vi "Convert_to_2009.vi"(8 "error in (no error)":errorcluster, 10 "2009 data in":T1={"DistSettings"={"BuildLabel"="", "ProductName"="", "BuildLocation"=path "", "MediaSize"=0, "Language"=9, "ProductVersion"={"Major"=1, "Minor"=0, "Update"=0}, "AutoIncrement"=FALSE, "ReadmeID"="", "LicenseID"="", "arpCompany"="", "arpURL"="http://", "arpContact"="", "arpPhone"="", "Executable"="", "CmdArg"="", "OSCheck"=0, "Hide"=FALSE, "LV80higher"=FALSE, "IncludeError?"=FALSE, "HWOption"=enum."<none>", "HWPath"=path "", "UpgradeCode"="", "Author"="", "MsiFileName"="", "CabFileName"="", "DistID"="", "WindowTitle"="", "WindowMessage"="", "CacheDistros"=FALSE, "EXE str ref?"=FALSE}, "BldInfo"=[], "FileInfo"=[], "DirInfo"=[], "ShortcutInfo"=[], "RegInfo"=[], "RegData"=[], "DistParts"=[], "DefaultDir"=""} {"RegData"."Values"."Type" items=["Bare", "String", "Expandable String", "Binary", "DWord"]; "DistSettings"."ProductVersion"."Update" step=1; "DistSettings"."ProductVersion"."Minor" step=1; "DistSettings"."ProductVersion"."Major" step=1; "DistSettings"."Language" items=["English"=9, "German"=7, "French"=12, "Japanese"=17, "Korean"=18, "Chinese (Simplified)"=2052]}, 11 "IB_Source_Build in":refnum<class "IB_Source_Build.lvclass">) -> (0 "error out":errorcluster, 2 "2009 data out":T1={"DistSettings"={"BuildLabel"="", "ProductName"="", "BuildLocation"=path "", "MediaSize"=0, "Language"=9, "ProductVersion"={"Major"=1, "Minor"=0, "Update"=0}, "AutoIncrement"=FALSE, "ReadmeID"="", "LicenseID"="", "arpCompany"="", "arpURL"="http://", "arpContact"="", "arpPhone"="", "Executable"="", "CmdArg"="", "OSCheck"=0, "Hide"=FALSE, "LV80higher"=FALSE, "IncludeError?"=FALSE, "HWOption"=enum."<none>", "HWPath"=path "", "UpgradeCode"="", "Author"="", "MsiFileName"="", "CabFileName"="", "DistID"="", "WindowTitle"="", "WindowMessage"="", "CacheDistros"=FALSE, "EXE str ref?"=FALSE}, "BldInfo"=[], "FileInfo"=[], "DirInfo"=[], "ShortcutInfo"=[], "RegInfo"=[], "RegData"=[], "DistParts"=[], "DefaultDir"=""} {"RegData"."Values"."Type" items=["Bare", "String", "Expandable String", "Binary", "DWord"]; "DistSettings"."ProductVersion"."Update" step=1; "DistSettings"."ProductVersion"."Minor" step=1; "DistSettings"."ProductVersion"."Major" step=1; "DistSettings"."Language" items=["English"=9, "German"=7, "French"=12, "Japanese"=17, "Korean"=18, "Chinese (Simplified)"=2052]})   [LabVIEW 2020, in "IB_Source_Build.lvclass"]
uses:
  <vilib>/AppBuilder/IB_Classes/Source/Container/Build/IB_Source_Build.lvclass
  <vilib>/AppBuilder/IB_Classes/Source/Container/Build/IB_Source_Build.lvclass/IB_Source_Build.ctl
  <vilib>/AppBuilder/IB_Classes/Source/IB_Source.lvclass
  <resource>/Framework/Providers/Builds/Installer/CDK_sTypeDef_BuildInfo.ctl
  <vilib>/AppBuilder/IB_Classes/Source/Container/IB_Source_Container.lvclass
  <resource>/Framework/Providers/Builds/Installer/CDK_sTypeDef_BuildTypes.ctl
  <vilib>/AppBuilder/IB_Classes/Source/File/IB_Source_File.lvclass
  e:/builds/penguin/labview/branches/2020/dev/dist/vi.lib/AppBuilder/IB_Classes/Source/Container/IB_Source_Container.lvclass
  e:/builds/penguin/labview/branches/2020/dev/dist/vi.lib/AppBuilder/IB_Classes/Source/IB_Source.lvclass
  e:/builds/penguin/labview/branches/2020/dev/dist/vi.lib/AppBuilder/IB_Classes/Source/Container/Build/IB_Source_Build.lvclass
  <vilib>/AppBuilder/IB_Classes/Source/File/CtrFile/IB_CtrFile.lvclass
  e:/builds/penguin/labview/branches/2020/dev/dist/vi.lib/AppBuilder/IB_Classes/Source/File/IB_Source_File.lvclass
  e:/builds/penguin/labview/branches/2020/dev/dist/vi.lib/AppBuilder/IB_Classes/Source/File/CtrFile/IB_CtrFile.lvclass
  <resource>/Framework/Providers/Builds/Installer/CDK_sTypeDef_FileInfo.ctl
  <resource>/Framework/Providers/Builds/Installer/CDK_sTypeDef_ShortcutInfo.ctl
  <resource>/Framework/Providers/Builds/Installer/CDK_sTypeDef_DirInfo.ctl
  <resource>/Framework/Providers/Builds/Installer/CDK_sTypeDef_Languages.ctl
  <resource>/Framework/Providers/Builds/Installer/CDK_sTypeDef_ProductVersion.ctl
  <resource>/Framework/Providers/Builds/Installer/CDK_sTypeDef_HWImportOption.ctl
  <resource>/Framework/Providers/Builds/Installer/CDK_sTypeDef_DISTSETTINGS.ctl
  AppLibs/distkit/MDF/NIMdf.llb/MDFBDPRegKeyType.ctl
  AppLibs/distkit/MDF/NI_MDF.lvlib
  <resource>/Framework/Providers/Builds/Installer/CDK_sTypeDef_RegData.ctl
  <resource>/Framework/Providers/Builds/Installer/CDK_sTypeDef_DistParts.ctl
  <vilib>/AppBuilder/IB_RW_Project/Compatibility/CDK_sTypeDef_2009_data.ctl
  <resource>/Framework/Providers/Builds/Installer/CDK_sTypeDef_SoftDep.ctl
panel:
  # "."
  # "."
  # "."
  # "."
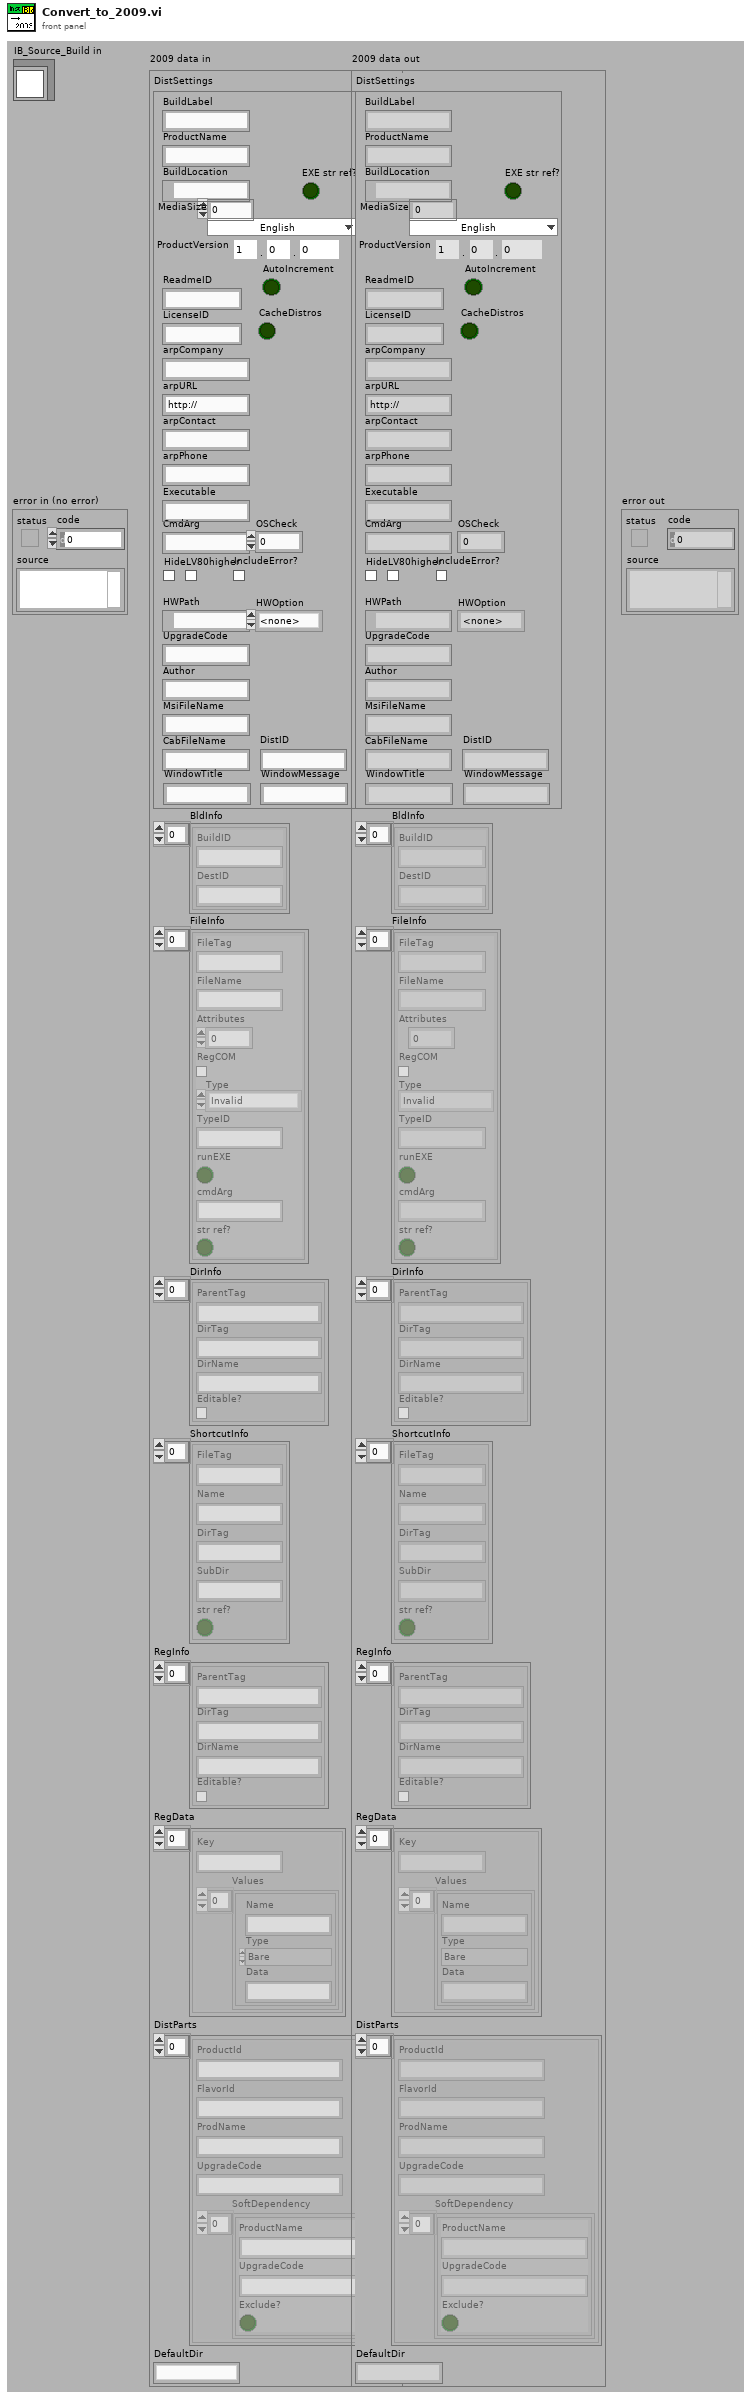
[diagram p1: front panel]
types:
  T1 = typedef "CDK_sTypeDef_2009_data.ctl" = cluster{"DistSettings":T2, "BldInfo":T6[], "FileInfo":T7[], "DirInfo":T9[], "ShortcutInfo":T10[], "RegInfo":T9[], "RegData":T11[], "DistParts":T13[], "DefaultDir":string}
  T2 = typedef "CDK_sTypeDef_DISTSETTINGS.ctl" = cluster{"BuildLabel":string, "ProductName":string, "BuildLocation":path, "MediaSize":u16, "Language":T3, "ProductVersion":T4, "AutoIncrement":bool, "ReadmeID":string, "LicenseID":string, "arpCompany":string, "arpURL":string, "arpContact":string, "arpPhone":string, "Executable":string, "CmdArg":string, "OSCheck":i32, "Hide":bool, "LV80higher":bool, "IncludeError?":bool, "HWOption":T5, "HWPath":path, "UpgradeCode":string, "Author":string, "MsiFileName":string, "CabFileName":string, "DistID":string, "WindowTitle":string, "WindowMessage":string, "CacheDistros":bool, "EXE str ref?":bool}
  T3 = typedef "CDK_sTypeDef_Languages.ctl" = u16
  T4 = typedef "CDK_sTypeDef_ProductVersion.ctl" = cluster{"Major":u8, "Minor":u8, "Update":u16}
  T5 = typedef "CDK_sTypeDef_HWImportOption.ctl" = enum16{"<none>", "Merge", "Replace", "Dialog"}
  T6 = typedef "CDK_sTypeDef_BuildInfo.ctl" = cluster{"BuildID":string, "DestID":string}
  T7 = typedef "CDK_sTypeDef_FileInfo.ctl" = cluster{"FileTag":string, "FileName":string, "Attributes":i16, "RegCOM":bool, "Type":T8, "TypeID":string, "runEXE":bool, "cmdArg":string, "str ref?":bool}
  T8 = typedef "CDK_sTypeDef_BuildTypes.ctl" = enum16{"Invalid", "File", "Folder", "BuildRule", "Library"}
  T9 = typedef "CDK_sTypeDef_DirInfo.ctl" = cluster{"ParentTag":string, "DirTag":string, "DirName":string, "Editable?":bool}
  T10 = typedef "CDK_sTypeDef_ShortcutInfo.ctl" = cluster{"FileTag":string, "Name":string, "DirTag":string, "SubDir":string, "str ref?":bool}
  T11 = typedef "CDK_sTypeDef_RegData.ctl" = cluster{"Key":string, "Values":cluster{"Name":string, "Type":T12, "Data":string}[]}
  T12 = typedef "NI_MDF.lvlib/MDFBDPRegKeyType.ctl" = i32
  T13 = typedef "CDK_sTypeDef_DistParts.ctl" = cluster{"ProductId":string, "FlavorId":string, "ProdName":string, "UpgradeCode":string, "SoftDependency":T14[]}
  T14 = typedef "CDK_sTypeDef_SoftDep.ctl" = cluster{"ProductName":string, "UpgradeCode":string, "Exclude?":bool}
  T15 = typedef "IB_Source.ctl" = cluster{"name":string, "sourceTag":string, "destTag":string, "path":path, "eng_installPath":string, "UI_inBuild?":bool, "str ref?":bool}
  T16 = typedef "IB_Source_Container.ctl" = cluster{"files":refnum<class "IB_CtrFile.lvclass">[], "previewed?":bool, "preview error?":bool}
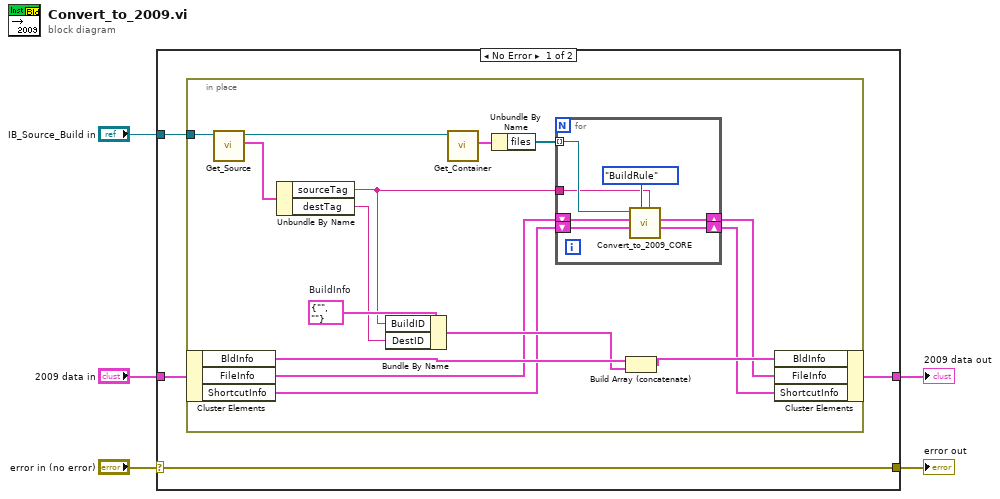
[diagram p0: block diagram]
diagram:
  n1 = case shown="No Error" "error in (no error)" {
    selector: "error in (no error)" -> [w9 w33]
    tunnel: [w9 w33] -> w4
    tunnel: "IB_Source_Build in" -> [w6 _]
    tunnel: "2009 data in" -> [w8 w32]
    tunnel: [w7 w32] -> w1
    frame No Error {
      n2 = in-place {
        in-place-border: w6 -> [w24]
        w20 = T6 {"BuildID"="", "DestID"=""}  # BuildInfo
        n3 = in-place-cluster #1(w8) -> ("BldInfo"=w22:T6[], "FileInfo"=w14:T7[], "ShortcutInfo"=w13:T10[])
        n4 = call <vilib>:"Get_Source.vi"("IB_Source in"=w24) -> ("data"=w23:T15, "IB_Source out"=w17:refnum<class "IB_Source_Build.lvclass">)  [unwired: 1 in, 8 out]
        n5 = Unbundle By Name(w23) -> ("sourceTag"=w10:string, "destTag"=w19:string)
        n6 = Bundle By Name(cluster=w20, "BuildID"=w10, "DestID"=w19) -> (w18:T6)
        n7 = call <vilib>:"Get_Container.vi"("IB_Source_Container in"=w17) -> ("data"=w16:T16)  [unwired: 1 in, 9 out]
        n8 = Unbundle By Name(w16) -> ("files"=w15:refnum<class "IB_CtrFile.lvclass">[])
        n9 = for {
          tunnel: w15 -> [w26] mode=indexing
          shift-right: [w30] -> w12
          shift-left: w14 -> [w28]
          shift-right: [w29] -> w11
          shift-left: w13 -> [w27]
          tunnel: w10 -> [w25]
          n10 = call <vilib>:"Convert_to_2009_CORE.vi"("TypeID"=w25, "Type"=CDK_sTypeDef_BuildTypes."BuildRule", "ShortcutInfoIn"=w27, "FileInfoIn"=w28, "IB_Source_File in"=w26) -> ("ShortcutInfoOut"=w29:T10[], "FileInfoOut"=w30:T7[])  [unwired: 2 in, 3 out]
        }
        n11 = Build Array (concatenate)(w22, w18) -> (w21:T6[])
        n12 = in-place-cluster #1("BldInfo"=w21, "FileInfo"=w12, "ShortcutInfo"=w11) -> (w7:T1)
      }
    }
    frame Error {
    }
  }
  "error out" <- w4
  "2009 data out" <- w1
